vi "DQMH-GenNet Set Network Info.vi"(6 "Timeout (default 5000ms)":i32=5000, 8 "error in (no error)":errorcluster, 9 "Port Number":u16, 10 "IP Address":string, 11 "Message Queue in":refnum<class "DQMH-GenNet Message Queue.lvclass">) -> (0 "error out":errorcluster, 3 "Message Queue out":refnum<class "DQMH-GenNet Message Queue.lvclass">)   [LabVIEW 2022 SP3, in "hse-gennet.lvlib" / "DQMH-GenNet Message Queue.lvclass"]
doc: "Sets or clears the network info in the Message Queue private data\n\n____\nHAMPEL SOFTWARE ENGINEERING v3.8.0 (2023-12-18 14:41)"
uses:
  DQMH-GenNet Message Queue.lvclass
  DQMH-GenNet Message Queue.lvclass/DQMH-GenNet Message Queue.ctl
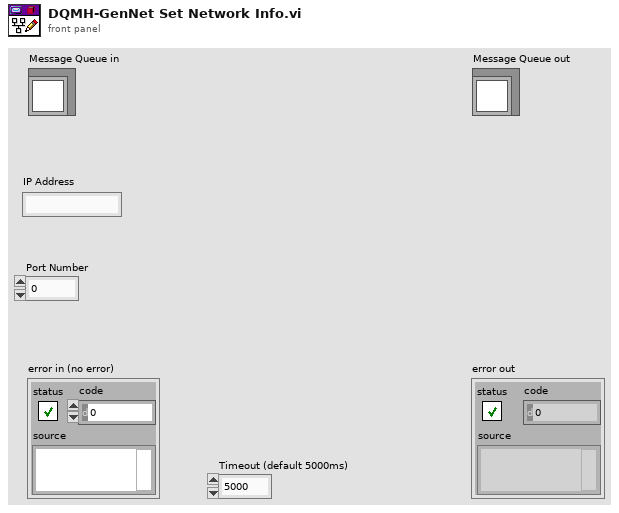
[diagram p1: front panel]
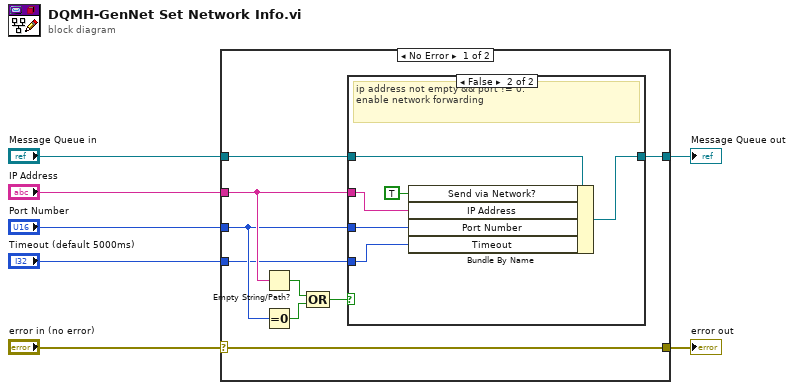
[diagram p0: block diagram]
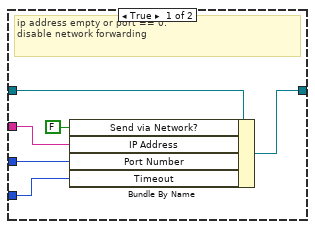
[diagram p2: hidden frame]
diagram:
  n1 = case shown="No Error" "error in (no error)" {
    selector: "error in (no error)" -> [w16 w29]
    tunnel: [w16 w29] -> w6
    tunnel: [w14 w30] -> w4
    tunnel: "Message Queue in" -> [w15 w30]
    tunnel: "IP Address" -> [w10 _]
    tunnel: "Port Number" -> [w9 _]
    tunnel: "Timeout (default 5000ms)" -> [w8 _]
    frame No Error {
      n2 = Empty String/Path?(string/path=w10) -> (empty?=w13:bool)
      n3 = Equal To 0?(x=w9) -> (x = 0?=w12:bool)
      n4 = Compound Arithmetic op=OR(w13, w12) -> (w11:bool)
      n5 = case shown="False" w11 {
        tunnel: w15 -> [w22 w28]
        tunnel: [w21 w27] -> w14
        tunnel: w10 -> [w19 w25]
        tunnel: w9 -> [w18 w24]
        tunnel: w8 -> [w17 w23]
        frame True {
          # "ip address empty or port == 0:\ndisable network forwarding"
          n6 = Bundle By Name(cluster=w22, "Send via Network?"=FALSE ("Networking.Send via Network?"), "IP Address"=w19, "Port Number"=w18, "Timeout"=w17) -> (w21:refnum<class "DQMH-GenNet Message Queue.lvclass">)
        }
        frame False {
          # "ip address not empty && port != 0:\nenable network forwarding"
          n7 = Bundle By Name(cluster=w28, "Send via Network?"=TRUE ("Networking.Send via Network?"), "IP Address"=w25, "Port Number"=w24, "Timeout"=w23) -> (w27:refnum<class "DQMH-GenNet Message Queue.lvclass">)
        }
      }
    }
    frame Error {
    }
  }
  "error out" <- w6
  "Message Queue out" <- w4
